vi "DataGridView.vi"() -> ()   [LabVIEW 2021]
uses:
  System.Windows.Forms
panel:
  out "error out":errorcluster
  out "Selection":string[](array[string])
  out "Count":i32
  in  "SelectionDone":bool
  in  "Elements":string[](array[string])
  out "Add":i32
  in  "DataGridView":refnum<k24>(container)
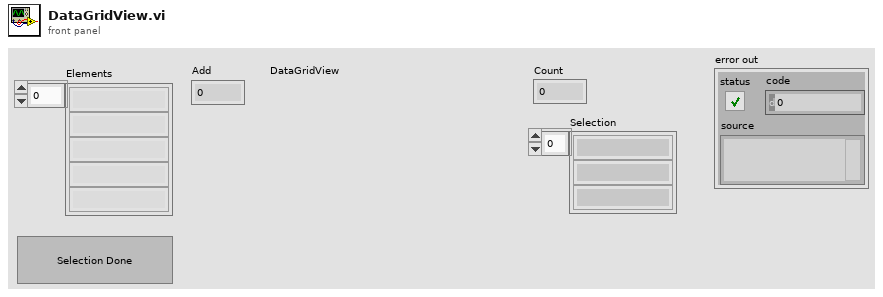
[diagram p1: front panel]
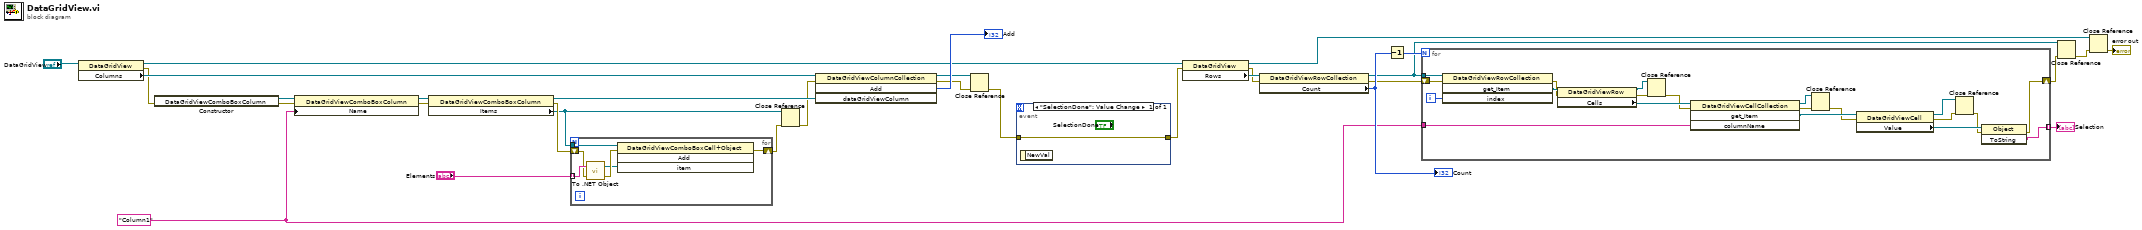
[diagram p0: block diagram]
diagram:
  w8 = "Column1" ("Name")
  n1 = property class="DataGridView"(reference="DataGridView") -> (reference out=w13:refnum<k24>, error out=w21:errorcluster, "Columns"=w31:refnum<k24>)  [unwired: 1 in]
  n2 = constructor class="DataGridViewComboBoxColumn"(error in=w21) -> (reference out=w28:refnum<k24>, error out=w24:errorcluster)  [unwired: 2 in, 1 out]
  n3 = property class="DataGridViewComboBoxColumn"(reference=w28, error in=w24, "Name"=w8) -> (reference out=w27:refnum<k24>, error out=w23:errorcluster)
  n4 = property class="DataGridViewComboBoxColumn"(reference=w27, error in=w23) -> (reference out=w26:refnum<k24>, error out=w22:errorcluster, "Items"=w17:refnum<k24>)
  n5 = for {
    tunnel: w17 -> [w37]
    tunnel: "Elements" -> [w35] mode=indexing
    shift-right: [w36] -> w16
    shift-left: w22 -> [w32]
    n6 = call <vilib>:"To .NET Object.vi"("error in (no error)"=w32, "anything"=w35) -> ("error out"=w34:errorcluster, ".NET object"=w33:refnum<k24>)
    n7 = invoke class="DataGridViewComboBoxCell+Object" method="Add"(reference=w37, error in=w34, "item"=w33) -> (error out=w36:errorcluster)  [unwired: 1 in, 3 out]
  }
  n8 = Close Reference(reference=w17, error in (no error)=w16) -> (error out=w15:errorcluster)
  n9 = invoke class="DataGridViewColumnCollection" method="Add"(reference=w31, error in=w15, "dataGridViewColumn"=w26) -> (reference out=w19:refnum<k24>, error out=w18:errorcluster, "Add"=→"Add":i32)  [unwired: 1 in, 1 out]
  n10 = Close Reference(reference=w19, error in (no error)=w18) -> (error out=w14:errorcluster)
  n11 = event shown="[0] \"SelectionDone\": Value Change" {
    selector: _ -> [_]
    dyn-events: _ -> [_]
    timeout: _ -> [_]
    tunnel: w14 -> [w38]
    tunnel: [w38] -> w20
    event "SelectionDone": Value Change {
      n12 = event-data() -> ()  [unwired: 1 in, 1 out]
    }
  }
  n13 = property class="DataGridView"(reference=w13, error in=w20) -> (reference out=w6:refnum<k24>, error out=w10:errorcluster, "Rows"=w12:refnum<k24>)
  n14 = property class="DataGridViewRowCollection"(reference=w12, error in=w10) -> (reference out=w3:refnum<k24>, error out=w9:errorcluster, "Count"=w11:i32)
  "Count" <- w11
  n15 = Decrement(x=w11) -> (x-1=w4:i32)
  n16 = for {
    N: w4 -> [_]
    tunnel: w3 -> [w58]
    shift-right: [w50] -> w2
    shift-left: w9 -> [w57]
    tunnel: w8 -> [w53]
    tunnel: [w49] -> w7 mode=indexing
    i -> [w56]
    n17 = invoke class="DataGridViewRowCollection" method="get_Item"(reference=w58, error in=w57, "index"=w56) -> (error out=w52:errorcluster, "get_Item"=w55:refnum<k24>)  [unwired: 1 in, 2 out]
    n18 = property class="DataGridViewRow"(reference=w55, error in=w52) -> (reference out=w41:refnum<k24>, error out=w40:errorcluster, "Cells"=w54:refnum<k24>)
    n19 = Close Reference(reference=w41, error in (no error)=w40) -> (error out=w39:errorcluster)
    n20 = invoke class="DataGridViewCellCollection" method="get_Item"(reference=w54, error in=w39, "columnName"=w53) -> (reference out=w45:refnum<k24>, error out=w43:errorcluster, "get_Item"=w44:refnum<k24>)  [unwired: 1 in, 1 out]
    n21 = Close Reference(reference=w45, error in (no error)=w43) -> (error out=w42:errorcluster)
    n22 = property class="DataGridViewCell"(reference=w44, error in=w42) -> (reference out=w48:refnum<k24>, error out=w47:errorcluster, "Value"=w51:refnum<k24>)
    n23 = Close Reference(reference=w48, error in (no error)=w47) -> (error out=w46:errorcluster)
    n24 = invoke class="Object" method="ToString"(reference=w51, error in=w46) -> (error out=w50:errorcluster, "ToString"=w49:string)  [unwired: 1 in, 1 out]
  }
  "Selection" <- w7
  n25 = Close Reference(reference=w3, error in (no error)=w2) -> (error out=w1:errorcluster)
  n26 = Close Reference(reference=w6, error in (no error)=w1) -> (error out=→"error out":errorcluster)
